vi "Tree To Trace.vi"(8 "Error In":errorcluster, 11 "Tree Control In":refnum<vi>) -> (0 "Error Out":errorcluster, 1 "Array":cluster{string, bool}[](array[cluster]), 3 "Tree Control Out":refnum<vi>)   [LabVIEW 2018, in "TraceTreeEditor.lvlib"]
uses:
  TraceTreeEditor.lvlib
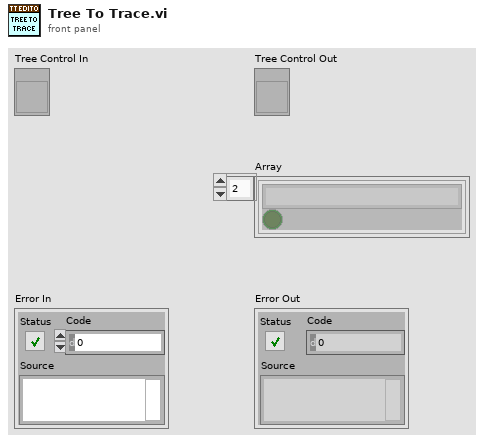
[diagram p1: front panel]
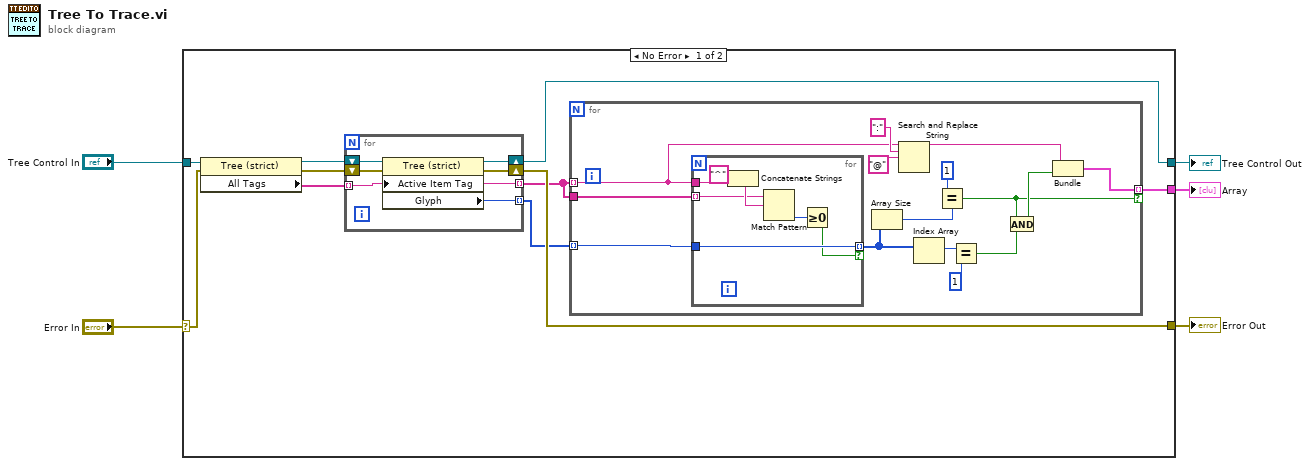
[diagram p0: block diagram]
diagram:
  n1 = case shown="No Error" "Error In" {
    selector: "Error In" -> [w15 w45]
    tunnel: "Tree Control In" -> [w11 w44]
    tunnel: [w9 _] -> w2
    tunnel: [w13 w45] -> w4
    tunnel: [w6 w44] -> w1
    frame No Error {
      n2 = property class="Tree (strict)"(reference=w11, error in=w15) -> (reference out=w12:refnum<vi>, error out=w14:errorcluster, "All Tags"=w10:string[])
      n3 = for {
        tunnel: w10 -> [w40] mode=indexing
        tunnel: [w40] -> w7 mode=indexing
        tunnel: [w39] -> w8 mode=indexing
        shift-right: [w38] -> w6
        shift-left: w12 -> [w41]
        shift-right: [w42] -> w13
        shift-left: w14 -> [w43]
        n4 = property class="Tree (strict)"(reference=w41, error in=w43, "Active Item Tag"=w40) -> (reference out=w38:refnum<vi>, error out=w42:errorcluster, "Glyph"=w39:i32)
      }
      n5 = for {
        tunnel: w7 -> [w16] mode=indexing
        tunnel: w8 -> [w30] mode=indexing
        tunnel: [w23] -> w9 mode=indexing if=w19
        tunnel: w7 -> [w17]
        n6 = for {
          tunnel: w16 -> [w35]
          tunnel: w30 -> [w36]
          tunnel: w17 -> [w32] mode=indexing
          tunnel: [w36] -> w27 mode=indexing if=w31
          n7 = Concatenate Strings("^" ("string"), w35) -> (w34:string)
          n8 = Match Pattern(string=w32, regular expression=w34) -> (offset past match=w37:i32)  [unwired: 1 in, 3 out]
          n9 = Greater Or Equal To 0?(x=w37) -> (x >= 0?=w31:bool)
        }
        n10 = Array Size(array=w27) -> (size(s)=w29:i32)
        n11 = Search and Replace String(input string=w16, search string=":", replace string="@" ("search string")) -> (result string=w22:string)  [unwired: 5 in, 3 out]
        n12 = Index Array(array=w27) -> (element=w26:i32)  [unwired: 1 in]
        n13 = Equal?(x=1, y=w29) -> (x = y?=w19:bool)
        n14 = Equal?(x=w26, y=1 ("x")) -> (x = y?=w18:bool)
        n15 = And(x=w19, y=w18) -> (x .and. y?=w24:bool)
        n16 = Bundle("result string"=w22, w24) -> (w23:cluster{"result string":string, bool})  [unwired: 1 in]
      }
    }
    frame Error {
    }
  }
  "Error Out" <- w4
  "Tree Control Out" <- w1
  "Array" <- w2
